vi "__uintCheckTimeout.vi"(1 "Millisecond timer value":u32, 2 "Timeout (-1)":T1) -> (0 "Timeout?":bool)   [LabVIEW 2011, in "UintClass.lvclass"]
uses:
  UintClass.lvclass
  timeout.ctl
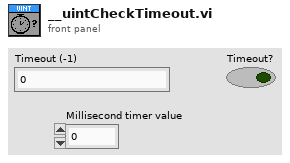
[diagram p1: front panel]
types:
  T1 = typedef "UintClass.lvclass/timeout.ctl" = i32
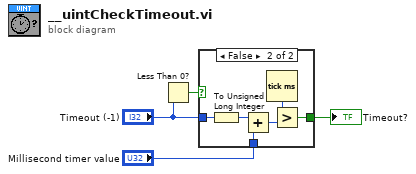
[diagram p0: block diagram]
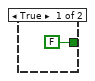
[diagram p2: hidden frame]
diagram:
  n1 = Less Than 0?(x="Timeout (-1)") -> (x < 0?=w1:bool)
  n2 = case shown="False" w1 {
    tunnel: "Millisecond timer value" -> [_ w11]
    tunnel: [FALSE w8] -> w4
    tunnel: "Timeout (-1)" -> [_ w6]
    frame True {
    }
    frame False {
      n3 = To Unsigned Long Integer(number=w6) -> (unsigned 32bit integer=w7:u32)
      n4 = Add(x=w7, y=w11) -> (x+y=w9:u32)
      n5 = Tick Count (ms)() -> (millisecond timer value=w10:u32)
      n6 = Greater?(x=w10, y=w9) -> (0:w8:bool)
    }
  }
  "Timeout?" <- w4
